vi "Schedule Build Nothing.vi"(6 "max geodes in":u8=24, 7 "max time in":u8=24, 8 "costs in":T1, 9 "data value reference":refnum<data-value>, 10 "stack in":refnum<queue>, 11 "mine in":refnum<class "Mine.lvclass">) -> (0 "costs out":T1, 1 "data value reference":refnum<data-value>, 2 "stack out":refnum<queue>, 3 "mine out":refnum<class "Mine.lvclass">, 4 "max geodes out":u8, 5 "max time out":u8)   [LabVIEW 2021, in "d19.lvlib" / "Mine.lvclass"]
uses:
  Mine.lvclass
  <vilib>/Utility/miscctls.llb/LVMapReplaceAction.ctl
  Mine.lvclass/Mine.ctl
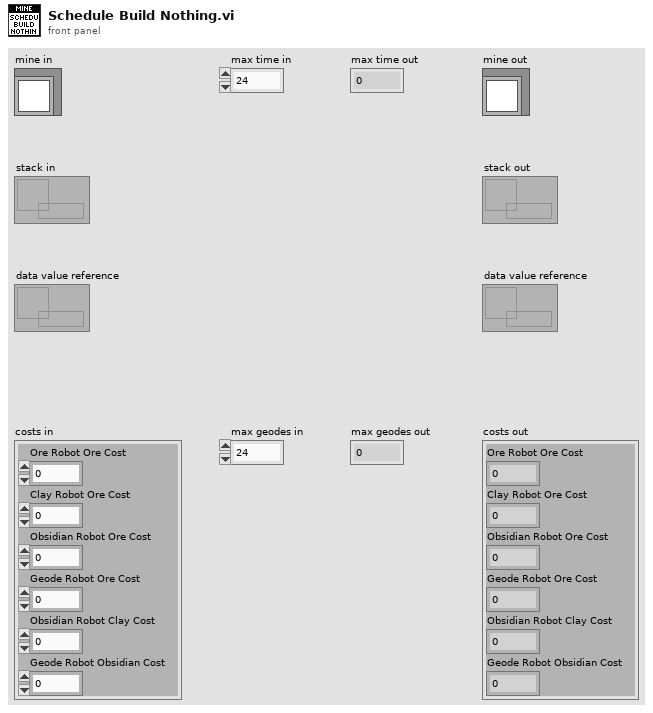
[diagram p1: front panel]
types:
  T1 = cluster{"Ore Robot Ore Cost":u8, "Clay Robot Ore Cost":u8, "Obsidian Robot Ore Cost":u8, "Geode Robot Ore Cost":u8, "Obsidian Robot Clay Cost":u8, "Geode Robot Obsidian Cost":u8}
  T2 = typedef "LVMapReplaceAction.ctl" = enum32{"Modify Entry only if found", "Add or Modify Entry", "Delete Entry"}
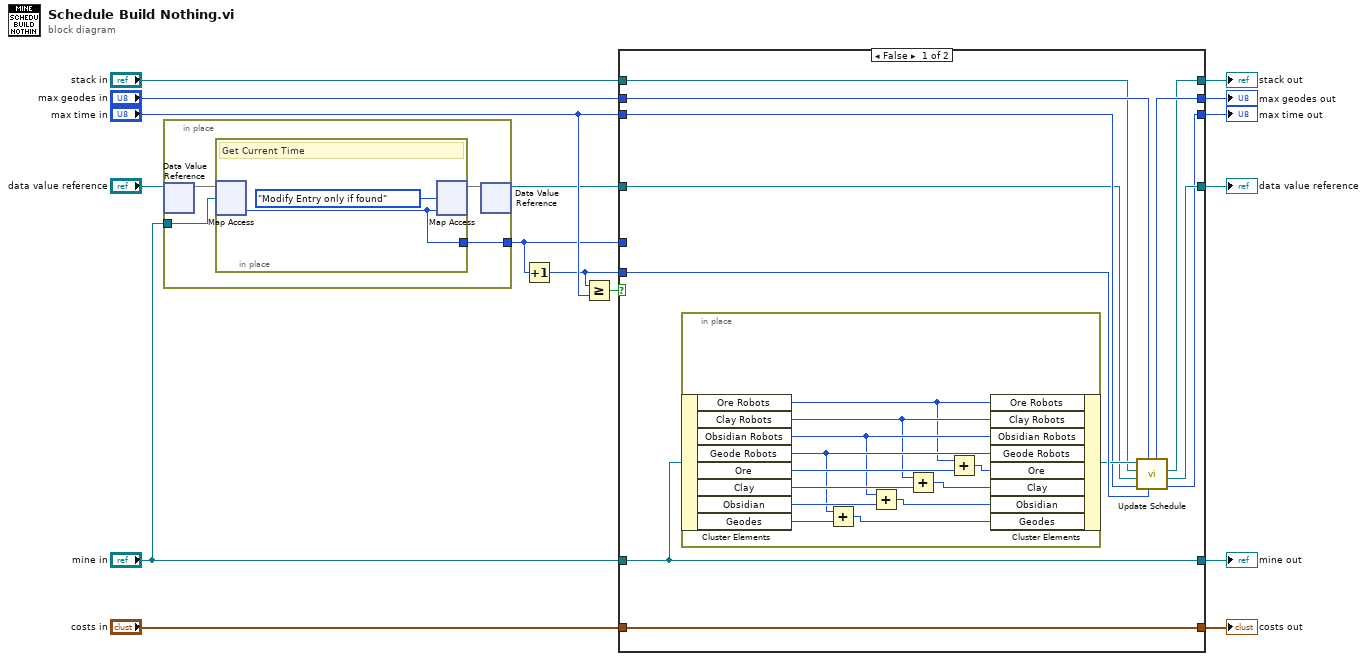
[diagram p0: block diagram]
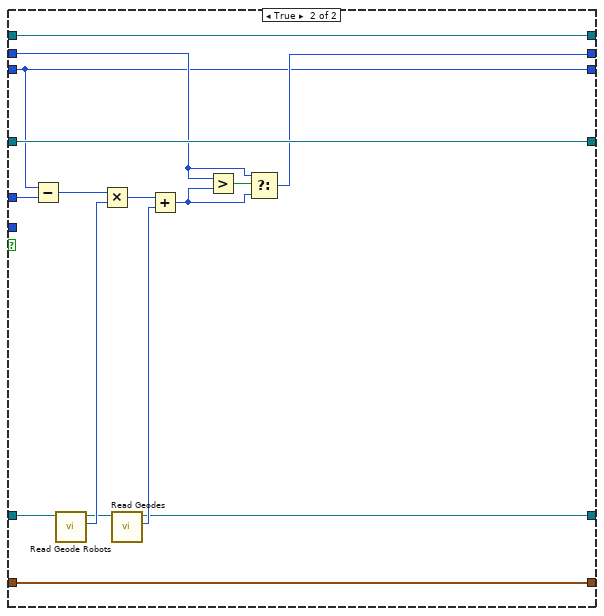
[diagram p2: hidden frame]
diagram:
  n1 = in-place {
    in-place-border: [w20] -> w5
    in-place-border: "mine in" -> [w17]
    n2 = in-place-dvr #1("data value reference") -> (w19:map{refnum<class "Mine.lvclass">, u8})  [unwired: 1 out]
    n3 = in-place {
      in-place-border: [w21] -> w20
      # "Get Current Time"
      n4 = in-place-map #2(w19, w17) -> (w21:u8)  [unwired: 1 in, 1 out]
      n5 = in-place-map #2(w21, LVMapReplaceAction."Modify Entry only if found" ("action")) -> (w18:map{refnum<class "Mine.lvclass">, u8})  [unwired: 2 out]
    }
    n6 = in-place-dvr #1(w18) -> (w6:refnum<data-value>)  [unwired: 1 out]
  }
  n7 = Increment(x=w5) -> (x+1=w4:u8)
  n8 = Greater Or Equal?(x=w4, y="max time in") -> (x >= y?=w1:bool)
  n9 = case shown="False" w1 {
    tunnel: w6 -> [w29 w62]
    tunnel: [w27 w62] -> w14
    tunnel: "stack in" -> [w28 w61]
    tunnel: [w26 w61] -> w15
    tunnel: "costs in" -> [w24 w60]
    tunnel: "mine in" -> [w23 w49]
    tunnel: [w24 w60] -> w13
    tunnel: [w23 w47] -> w12
    tunnel: "max time in" -> [w30 w56]
    tunnel: w5 -> [_ w55]
    tunnel: "max geodes in" -> [w34 w57]
    tunnel: [w33 w58] -> w9
    tunnel: [w25 w56] -> w8
    tunnel: w4 -> [w32 _]
    frame False {
      n10 = in-place {
        n11 = in-place-cluster #3(w23) -> ("Ore Robots"=w35:u8, "Clay Robots"=w36:u8, "Obsidian Robots"=w37:u8, "Geode Robots"=w38:u8, "Ore"=w46:u8, "Clay"=w44:u8, "Obsidian"=w41:u8, "Geodes"=w43:u8)
        n12 = Add(x=w38, y=w43) -> (x+y=w39:u8)
        n13 = Add(x=w37, y=w41) -> (x+y=w40:u8)
        n14 = Add(x=w36, y=w44) -> (x+y=w42:u8)
        n15 = Add(x=w35, y=w46) -> (x+y=w45:u8)
        n16 = in-place-cluster #3("Ore Robots"=w35, "Clay Robots"=w36, "Obsidian Robots"=w37, "Geode Robots"=w38, "Ore"=w45, "Clay"=w42, "Obsidian"=w40, "Geodes"=w39) -> (w31:refnum<class "Mine.lvclass">)
      }
      n17 = call "Update Schedule.vi"("new time"=w32, "max geodes in"=w34, "max time in"=w30, "map in"=w29, "stack in"=w28, "Mine in"=w31) -> ("max time out"=w25:u8, "map out"=w27:refnum<data-value>, "stack out"=w26:refnum<queue>, "max geodes out"=w33:u8)  [unwired: 1 in, 1 out]
    }
    frame True {
      n18 = Subtract(x=w56, y=w55) -> (x-y=w54:u8)
      n19 = call "Read Geode Robots.vi"("Mine in"=w49) -> ("Geode Robots"=w53:u8, "Mine out"=w48:refnum<class "Mine.lvclass">)  [unwired: 9 in]
      n20 = Multiply(x=w54, y=w53) -> (x*y=w50:u8)
      n21 = call "Read Geodes.vi"("Mine in"=w48) -> ("Geodes"=w52:u8, "Mine out"=w47:refnum<class "Mine.lvclass">)  [unwired: 9 in]
      n22 = Add(x=w50, y=w52) -> (x+y=w51:u8)
      n23 = Greater?(x=w57, y=w51) -> (0:w59:bool)
      n24 = Select(t=w57, s=w59, f=w51) -> (s? t:f=w58:u8)
    }
  }
  "stack out" <- w15
  "data value reference" <- w14
  "costs out" <- w13
  "mine out" <- w12
  "max geodes out" <- w9
  "max time out" <- w8
